vi "Angle Distance.vi"(1 "Target Angle":dbl(knob) scale=-180.0..180.0, 2 "Current Angle":dbl(knob) scale=-180.0..180.0) -> (0 "Distance":dbl)   [LabVIEW 2016]
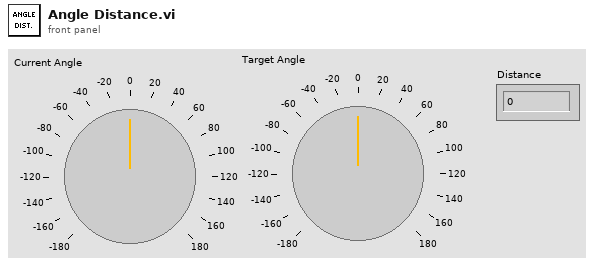
[diagram p1: front panel]
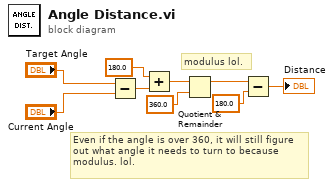
[diagram p0: block diagram]
diagram:
  # "Even if the angle is over 360, it will still figure\nout what angle it needs to turn to because \nmodulus. lol."
  # "modulus lol."
  n1 = Subtract(x="Target Angle", y="Current Angle") -> (x-y=w7:dbl)
  n2 = Add(x=180.0, y=w7) -> (x+y=w5:dbl)
  n3 = Quotient & Remainder(x=w5, y=360.0) -> (x-y*floor(x/y)=w3:dbl)  [unwired: 1 out]
  n4 = Subtract(x=w3, y=180.0) -> (x-y=→"Distance":dbl)
